vi "Write ILC.vi"(10 "ILC":refnum<class "ILC.lvclass">, 11 "IILCDAC in":refnum<class "IILCDAC.lvclass">) -> (3 "IILCDAC out":refnum<class "IILCDAC.lvclass">)   [LabVIEW 2015]
uses:
  IILCDAC.lvclass
  <userlib>/Common/ILC/ILC/ILC.lvclass
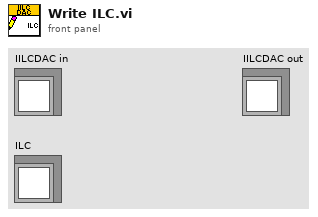
[diagram p1: front panel]
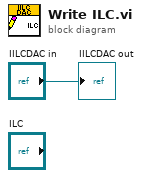
[diagram p0: block diagram]
diagram:
  "IILCDAC out" <- "IILCDAC in"
